vi "Measurement Logic.vi"() -> ()   [LabVIEW 2021, in "Sweep_Channel Ganging.lvlib"]
uses:
  Sweep_Channel Ganging.lvlib
  Measurement Results.ctl
  <vilib>/Plug-In SDKs/Measurements/Measure Call Context/Measure Call Context.lvclass
  Measurement Configuration.ctl
  shared/Ganging/controls/Power ON-Ganging.ctl
  shared/Single/controls/Power ON-Single.ctl
panel:
  in  "measurement configuration":T1={"Mode of operation"=enum."Power on the DUT", "Source enable/disable"=TRUE, "Load enable/disable"=TRUE, "Source resource names"=[], "Load resource names"=[], "Power ON/Source system configuration"=enum."Parallel", "Power ON/Source output function"=1006, "Source sweep scale"="Linear", "Power ON V/I Source start level"=6.0, "Source stop level"=20.0, "Source sweep points/points per decade"=4, "Source voltage/current level range"=20.0, "Power ON/Source sense"=1009, "Source limit symmetry"=enum."Asymmetric", "Power ON/Source current/voltage limit range"=25.0, "Source current/voltage limit low"=-0.6, "Source current/voltage limit high"=25.0, "Source source delay"=0.005, "Source aperture time"=0.01666, "Source transient response"=1038, "Source voltage/current gain bandwidth"=2000.0, "Source voltage/current compensation frequency"=3530.0, "Source voltage/current pole-zero ratio"=2.0, "Load system configuration"=enum."Parallel", "Load output function"=1007, "Load device voltage/current rating"=50.0, "Load sweep scale"="Linear", "Load start level"=1.0, "Load stop level"=50.0, "Load sweep points/points per decade"=10, "Load voltage/current level range"=80.0, "Load sense"=1009, "Load limit symmetry"=enum."Symmetric", "Load current/voltage limit range"=6.0, "Load current/voltage limit low"=0.0, "Load current/voltage limit high"=inf, "Load source delay"=0.005, "Load aperture time"=0.01666, "Load transient response"=1038, "Load voltage/current gain bandwidth"=10000.0, "Load voltage/current compensation frequency"=50000.0, "Load voltage/current pole-zero ratio"=12.0, "Load source trigger"="", "Load measure trigger"="", "Measurement timeout"=10.0} {"Measurement timeout" format="%.3p"; "Load device voltage/current rating" format="%#_6pA"; "Load output function" items=["DC Voltage"=1006, "DC Current"=1007, "Pulse Voltage"=1049, "Pulse Current"=1050]; "Power ON/Source output function" items=["DC Voltage"=1006, "DC Current"=1007, "Pulse Voltage"=1049, "Pulse Current"=1050]; "Load sweep points/points per decade" format="%#_6p"; "Power ON V/I Source start level" format="%#_6p"; "Load sense" items=["Symmetric", "Asymmetric"]; "Load transient response" items=["Slow"=1041, "Normal"=1038, "Fast"=1039, "Custom"=1042]; "Power ON/Source sense" items=["Local"=1008, "Remote"=1009]; "Source transient response" items=["Slow"=1041, "Normal"=1038, "Fast"=1039, "Custom"=1042]; "Load current/voltage limit low" format="%#_6p"; "Load current/voltage limit range" format="%#_6p"; "Load voltage/current level range" format="%#_6p"; "Source current/voltage limit high" format="%#_6p"; "Source current/voltage limit low" format="%#_6p"; "Power ON/Source current/voltage limit range" format="%#_6p"; "Source voltage/current level range" format="%#_6p"}
  in  "error in":errorcluster
  out "measure call context out":refnum<class "Measure Call Context.lvclass">
  in  "measure call context in":refnum<class "Measure Call Context.lvclass">
  out "measurement results":T2
  out "error out":errorcluster
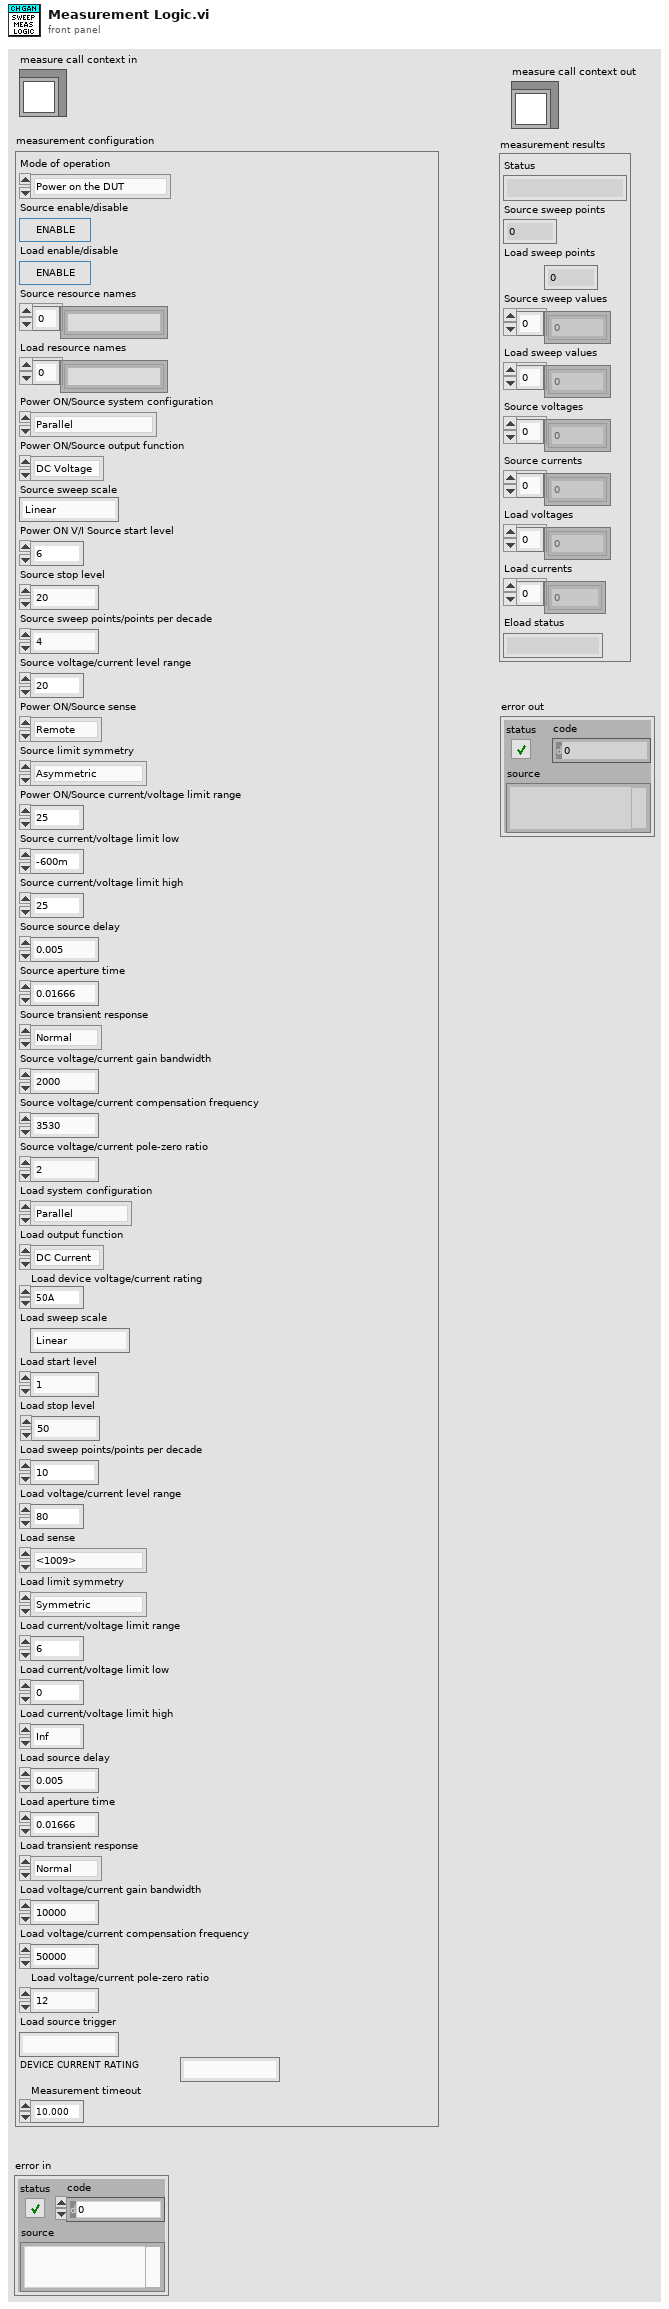
[diagram p1: front panel]
types:
  T1 = typedef "Sweep_Channel Ganging.lvlib/Measurement Configuration.ctl" = cluster{"Mode of operation":enum32{"Power on the DUT", "Perform measurement", "Power off the DUT"}, "Source enable/disable":bool, "Load enable/disable":bool, "Source resource names":string[], "Load resource names":string[], "Power ON/Source system configuration":enum32{"Series", "Parallel", "Manual"}, "Power ON/Source output function":i32, "Source sweep scale":string, "Power ON V/I Source start level":dbl, "Source stop level":dbl, "Source sweep points/points per decade":i32, "Source voltage/current level range":dbl, "Power ON/Source sense":i32, "Source limit symmetry":enum32{"Symmetric", "Asymmetric"}, "Power ON/Source current/voltage limit range":dbl, "Source current/voltage limit low":dbl, "Source current/voltage limit high":dbl, "Source source delay":dbl, "Source aperture time":dbl, "Source transient response":i32, "Source voltage/current gain bandwidth":dbl, "Source voltage/current compensation frequency":dbl, "Source voltage/current pole-zero ratio":dbl, "Load system configuration":enum32{"Series", "Parallel", "Manual"}, "Load output function":i32, "Load device voltage/current rating":dbl, "Load sweep scale":string, "Load start level":dbl, "Load stop level":dbl, "Load sweep points/points per decade":i32, "Load voltage/current level range":dbl, "Load sense":i32, "Load limit symmetry":enum32{"Symmetric", "Asymmetric"}, "Load current/voltage limit range":dbl, "Load current/voltage limit low":dbl, "Load current/voltage limit high":dbl, "Load source delay":dbl, "Load aperture time":dbl, "Load transient response":i32, "Load voltage/current gain bandwidth":dbl, "Load voltage/current compensation frequency":dbl, "Load voltage/current pole-zero ratio":dbl, "Load source trigger":string, "Load measure trigger":string, "Measurement timeout":dbl}
  T2 = typedef "Sweep_Channel Ganging.lvlib/Measurement Results.ctl" = cluster{"Status":string, "Source sweep points":i32, "Load sweep points":i32, "Source sweep values":dbl[], "Load sweep values":dbl[], "Source voltages":dbl[], "Source currents":dbl[], "Load voltages":dbl[], "Load currents":dbl[], "Eload status":string}
  T3 = enum32{"Power on the DUT", "Perform measurement", "Power off the DUT"}
  T4 = typedef "Power ON-Ganging.ctl" = cluster{"Master/single Resource name":string, "Slave resource name":string[], "System configuration":enum32{"Series", "Parallel", "Manual"}, "Output function":i32, "Voltage/current level":dbl, "Voltage/current limit":dbl, "Sense":i32}
  T5 = typedef "Power ON-Single.ctl" = cluster{"Voltage/current level":dbl, "Voltage/current limit":dbl, "Sense":i32, "Resource name":string, "Output function":i32}
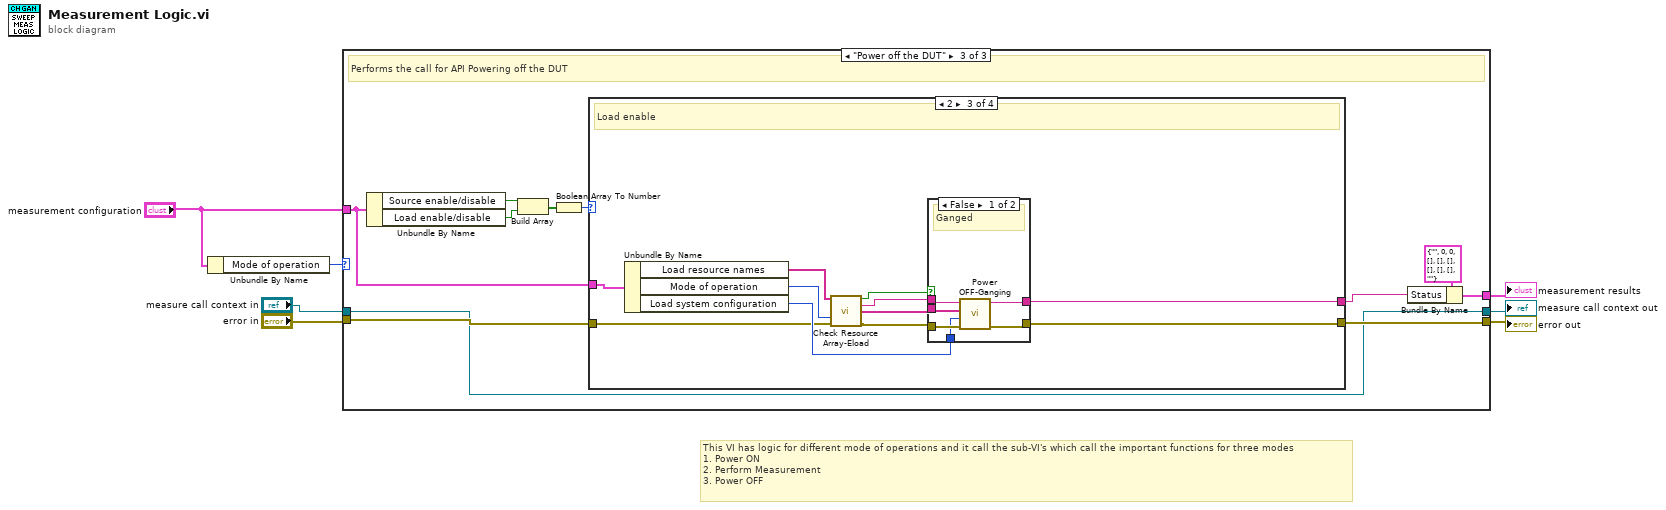
[diagram p0: block diagram]
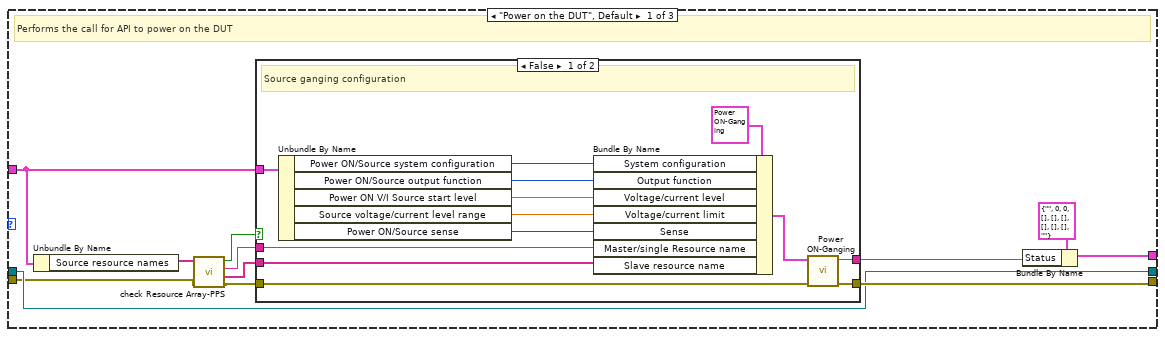
[diagram p2: hidden frame]
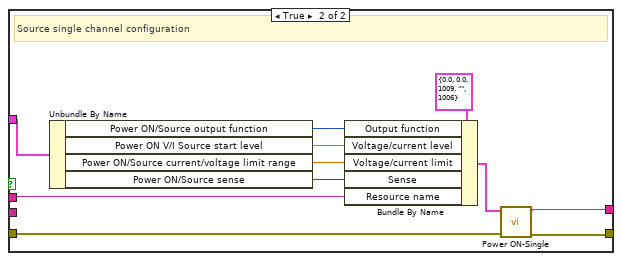
[diagram p3: hidden frame]
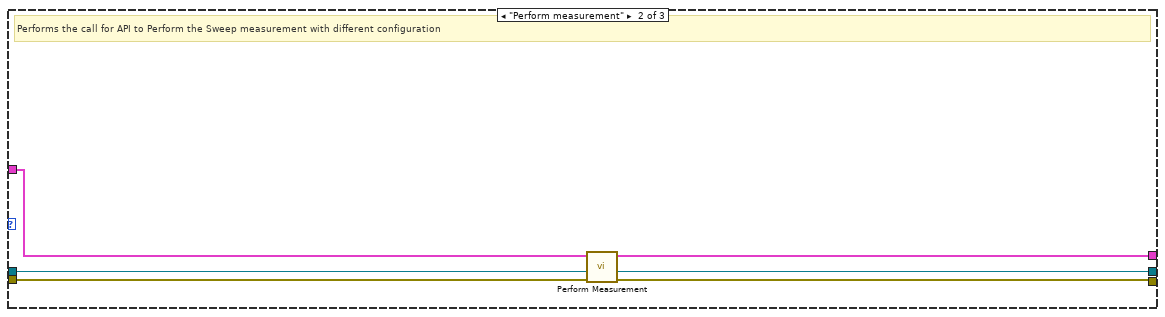
[diagram p4: hidden frame]
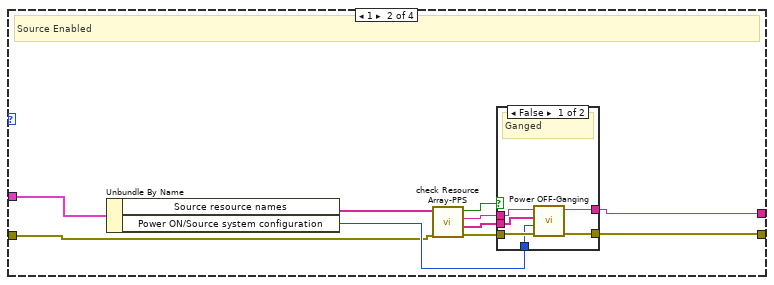
[diagram p6: hidden frame]
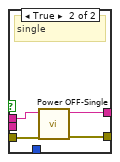
[diagram p7: hidden frame]
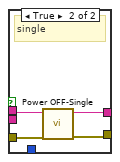
[diagram p8: hidden frame]
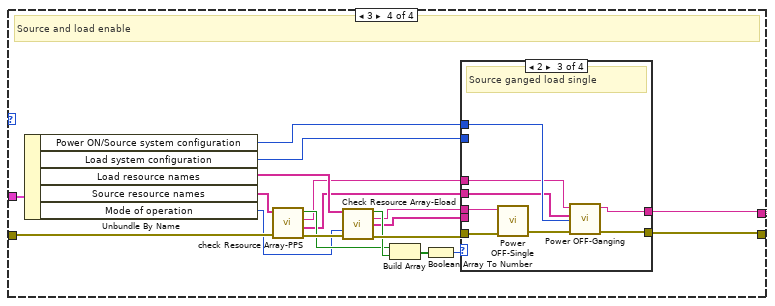
[diagram p9: hidden frame]
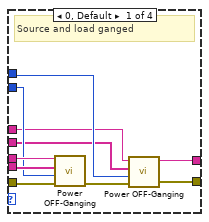
[diagram p10: hidden frame]
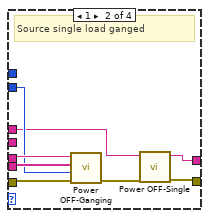
[diagram p11: hidden frame]
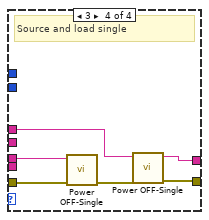
[diagram p12: hidden frame]
diagram:
  # "This VI has logic for different mode of operations and it call the sub-VI's which call the important functions for three modes\n1. Power ON\n2. Perform Measurement\n3. Power OFF"
  n1 = Unbundle By Name("measurement configuration") -> ("Mode of operation"=w5:T3)
  n2 = case shown="\"Power off the DUT\"" w5 {
    tunnel: [w19 w49 w54] -> w7
    tunnel: "error in" -> [w16 w44 w56]
    tunnel: "measurement configuration" -> [w18 w47 w55]
    tunnel: "measure call context in" -> [w17 w48 w53]
    tunnel: [w17 w45 w53] -> w3
    tunnel: [w9 w46 w50] -> w1
    frame "Power on the DUT", Default {
      # "Performs the call for API to power on the DUT"
      n3 = Unbundle By Name(w18) -> ("Source resource names"=w12:string[])
      n4 = call "check Resource Array-PPS.vi"("error in"=w16, "Resource names"=w12) -> ("error out"=w15:errorcluster, "Slave resource names"=w13:string[], "Single/Master resouce names"=w14:string, "Single or ganged configuration"=w11:bool)  [unwired: 6 in]
      n5 = case shown="False" w11 {
        tunnel: w15 -> [w24 w39]
        tunnel: [w25 w38] -> w19
        tunnel: w13 -> [w30 _]
        tunnel: w18 -> [w32 w43]
        tunnel: w14 -> [w31 w34]
        tunnel: [w26 w37] -> w8
        frame False {
          # "Source ganging configuration"
          n6 = Unbundle By Name(w32) -> ("Power ON/Source system configuration"=w23:enum32{"Series", "Parallel", "Manual"}, "Power ON/Source output function"=w22:i32, "Power ON V/I Source start level"=w29:dbl, "Source voltage/current level range"=w28:dbl, "Power ON/Source sense"=w27:i32)
          n7 = Bundle By Name(cluster=T4 {"Master/single Resource name"="", "Slave resource name"=[], "System configuration"=enum."Parallel", "Output function"=1006, "Voltage/current level"=0.0, "Voltage/current limit"=0.0, "Sense"=1009} ("Power ON"), "System configuration"=w23, "Output function"=w22, "Voltage/current level"=w29, "Voltage/current limit"=w28, "Sense"=w27, "Master/single Resource name"=w31, "Slave resource name"=w30) -> (w20:T4)
          n8 = call "Power ON-Ganging.vi"("error in"=w24, "Power ON"=w20) -> ("error out"=w25:errorcluster, "Status"=w26:string)  [unwired: 8 in]
        }
        frame True {
          # "Source single channel configuration"
          n9 = Unbundle By Name(w43) -> ("Power ON/Source output function"=w36:i32, "Power ON V/I Source start level"=w40:dbl, "Power ON/Source current/voltage limit range"=w41:dbl, "Power ON/Source sense"=w42:i32)
          n10 = Bundle By Name(cluster=T5 {"Voltage/current level"=0.0, "Voltage/current limit"=0.0, "Sense"=1009, "Resource name"="", "Output function"=1006} ("Power ON single"), "Output function"=w36, "Voltage/current level"=w40, "Voltage/current limit"=w41, "Sense"=w42, "Resource name"=w34) -> (w35:T5)
          n11 = call "Power ON-Single.vi"("error in"=w39, "Power ON single"=w35) -> ("error out"=w38:errorcluster, "Status"=w37:string)  [unwired: 8 in]
        }
      }
      n12 = Bundle By Name(cluster=T2 {"Status"="", "Source sweep points"=0, "Load sweep points"=0, "Source sweep values"=[], "Load sweep values"=[], "Source voltages"=[], "Source currents"=[], "Load voltages"=[], "Load currents"=[], "Eload status"=""} ("measurement results"), "Status"=w8) -> (w9:T2)
    }
    frame "Perform measurement" {
      # "Performs the call for API to Perform the Sweep measurement with different configuration"
      n13 = call "Perform Measurement.vi"("error in (no error)"=w44, "Measure Call Context in"=w48, "measurement configuration"=w47) -> ("error out"=w49:errorcluster, "Measure Call Context out"=w45:refnum<class "Measure Call Context.lvclass">, "Measurement Results"=w46:T2)  [unwired: 5 in]
    }
    frame "Power off the DUT" {
      # "Performs the call for API Powering off the DUT"
      n14 = Unbundle By Name(w55) -> ("Source enable/disable"=w60:bool, "Load enable/disable"=w59:bool)
      n15 = Build Array(w60, w59) -> (w58:bool[])
      n16 = Boolean Array To Number(Boolean array=w58) -> (number=w57:u32)
      n17 = case shown="2" w57 {
        tunnel: w55 -> [_ w71 w92 w121]
        tunnel: w56 -> [w61 w66 w88 w109]
        tunnel: [w61 w70 w91 w118] -> w54
        tunnel: [_ w68 w90 w117] -> w51
        frame 0, Default {
          # "Source and load off"
        }
        frame 1 {
          # "Source Enabled"
          n18 = Unbundle By Name(w71) -> ("Source resource names"=w67:string[], "Power ON/Source system configuration"=w69:enum32{"Series", "Parallel", "Manual"})
          n19 = call "check Resource Array-PPS.vi"("error in"=w66, "Resource names"=w67) -> ("error out"=w65:errorcluster, "Slave resource names"=w62:string[], "Single/Master resouce names"=w63:string, "Single or ganged configuration"=w64:bool)  [unwired: 6 in]
          n20 = case shown="False" w64 {
            tunnel: w65 -> [w77 w79]
            tunnel: [w72 w80] -> w70
            tunnel: [w76 w81] -> w68
            tunnel: w69 -> [w75 _]
            tunnel: w63 -> [w74 w78]
            tunnel: w62 -> [w73 _]
            frame False {
              # "Ganged"
              n21 = call "Power OFF-Ganging.vi"("error in"=w77, "Ganged Config"=w75, "Slave resource names"=w73, "Master resouce name"=w74) -> ("error out"=w72:errorcluster, "Status"=w76:string)  [unwired: 6 in]
            }
            frame True {
              # "single"
              n22 = call "Power OFF-Single.vi"("error in (no error)"=w79, "Resource name"=w78) -> ("error out"=w80:errorcluster, "Status"=w81:string)  [unwired: 8 in]
            }
          }
        }
        frame 2 {
          # "Load enable"
          n23 = Unbundle By Name(w92) -> ("Load resource names"=w83:string[], "Mode of operation"=w82:T3, "Load system configuration"=w89:enum32{"Series", "Parallel", "Manual"})
          n24 = call "Check Resource Array-Eload.vi"("Resource names"=w83, "Mode of operation"=w82, "error in"=w88) -> ("Single or ganged configuration"=w86:bool, "Single/Master resouce name"=w85:string, "Slave resource names"=w84:string[], "error out"=w87:errorcluster)  [unwired: 8 in, 1 out]
          n25 = case shown="False" w86 {
            tunnel: w87 -> [w98 w101]
            tunnel: [w93 w99] -> w91
            tunnel: [w97 w100] -> w90
            tunnel: w85 -> [w96 w102]
            tunnel: w84 -> [w95 _]
            tunnel: w89 -> [w94 _]
            frame False {
              # "Ganged"
              n26 = call "Power OFF-Ganging.vi"("error in"=w98, "Ganged Config"=w94, "Slave resource names"=w95, "Master resouce name"=w96) -> ("error out"=w93:errorcluster, "Status"=w97:string)  [unwired: 6 in]
            }
            frame True {
              # "single"
              n27 = call "Power OFF-Single.vi"("error in (no error)"=w101, "Resource name"=w102) -> ("error out"=w99:errorcluster, "Status"=w100:string)  [unwired: 8 in]
            }
          }
        }
        frame 3 {
          # "Source and load enable"
          n28 = Unbundle By Name(w121) -> ("Power ON/Source system configuration"=w115:enum32{"Series", "Parallel", "Manual"}, "Load system configuration"=w116:enum32{"Series", "Parallel", "Manual"}, "Load resource names"=w110:string[], "Source resource names"=w107:string[], "Mode of operation"=w103:T3)
          n29 = call "check Resource Array-PPS.vi"("error in"=w109, "Resource names"=w107) -> ("error out"=w108:errorcluster, "Slave resource names"=w104:string[], "Single/Master resouce names"=w105:string, "Single or ganged configuration"=w106:bool)  [unwired: 6 in]
          n30 = call "Check Resource Array-Eload.vi"("Resource names"=w110, "Mode of operation"=w103, "error in"=w108) -> ("Single or ganged configuration"=w113:bool, "Single/Master resouce name"=w112:string, "Slave resource names"=w111:string[], "error out"=w114:errorcluster)  [unwired: 8 in, 1 out]
          n31 = Build Array(w106, w113) -> (w120:bool[])
          n32 = Boolean Array To Number(Boolean array=w120) -> (number=w119:u32)
          n33 = case shown="2" w119 {
            tunnel: w114 -> [w130 w139 w147 w153]
            tunnel: [w122 w137 w140 w151] -> w118
            tunnel: [w131 w138 w143 w149] -> w117
            tunnel: w112 -> [w129 w136 w146 w150]
            tunnel: w111 -> [w128 w135 _ _]
            tunnel: w116 -> [w127 w134 _ _]
            tunnel: w115 -> [w126 _ w144 _]
            tunnel: w105 -> [w124 w133 w142 w148]
            tunnel: w104 -> [w125 _ w141 _]
            frame 0, Default {
              # "Source and load ganged"
              n34 = call "Power OFF-Ganging.vi"("error in"=w130, "Ganged Config"=w127, "Slave resource names"=w128, "Master resouce name"=w129) -> ("error out"=w123:errorcluster)  [unwired: 6 in, 1 out]
              n35 = call "Power OFF-Ganging.vi"("error in"=w123, "Ganged Config"=w126, "Slave resource names"=w125, "Master resouce name"=w124) -> ("error out"=w122:errorcluster, "Status"=w131:string)  [unwired: 6 in]
            }
            frame 1 {
              # "Source single load ganged"
              n36 = call "Power OFF-Ganging.vi"("error in"=w139, "Ganged Config"=w134, "Slave resource names"=w135, "Master resouce name"=w136) -> ("error out"=w132:errorcluster)  [unwired: 6 in, 1 out]
              n37 = call "Power OFF-Single.vi"("error in (no error)"=w132, "Resource name"=w133) -> ("error out"=w137:errorcluster, "Status"=w138:string)  [unwired: 8 in]
            }
            frame 2 {
              # "Source ganged load single"
              n38 = call "Power OFF-Single.vi"("error in (no error)"=w147, "Resource name"=w146) -> ("error out"=w145:errorcluster)  [unwired: 8 in, 1 out]
              n39 = call "Power OFF-Ganging.vi"("error in"=w145, "Ganged Config"=w144, "Slave resource names"=w141, "Master resouce name"=w142) -> ("error out"=w140:errorcluster, "Status"=w143:string)  [unwired: 6 in]
            }
            frame 3 {
              # "Source and load single"
              n40 = call "Power OFF-Single.vi"("error in (no error)"=w153, "Resource name"=w150) -> ("error out"=w152:errorcluster)  [unwired: 8 in, 1 out]
              n41 = call "Power OFF-Single.vi"("error in (no error)"=w152, "Resource name"=w148) -> ("error out"=w151:errorcluster, "Status"=w149:string)  [unwired: 8 in]
            }
          }
        }
      }
      n42 = Bundle By Name(cluster=T2 {"Status"="", "Source sweep points"=0, "Load sweep points"=0, "Source sweep values"=[], "Load sweep values"=[], "Source voltages"=[], "Source currents"=[], "Load voltages"=[], "Load currents"=[], "Eload status"=""} ("measurement results"), "Status"=w51) -> (w50:T2)
    }
  }
  "error out" <- w7
  "measurement results" <- w1
  "measure call context out" <- w3
